vi "Parse NT String Array.vi"(11 "TCP Network Connection in":refnum<k5>) -> (1 "Size":i32=1, 2 "String Array":string[](array[string]), 3 "TCP Network Connection out":refnum<k5>)   [LabVIEW 2017]
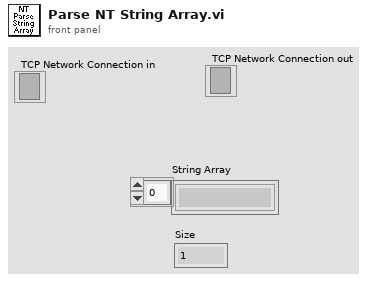
[diagram p1: front panel]
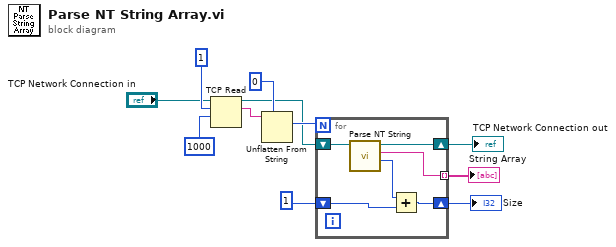
[diagram p0: block diagram]
diagram:
  n1 = TCP Read(connection ID="TCP Network Connection in", bytes to read=1 ("timeout ms (25000)"), 9:1000 ("timeout ms (25000)")) -> (connection ID out=w5:refnum<k5>, data out=w8:string)  [unwired: 2 in, 1 out]
  n2 = Unflatten From String(type=u8 0 ("Size"), binary string=w8) -> (value=w6:u8)  [unwired: 3 in, 2 out]
  n3 = for {
    N: w6 -> [_]
    shift-right: [w16] -> w4
    shift-left: w5 -> [w17]
    tunnel: [w15] -> w3 mode=indexing
    shift-right: [w13] -> w1
    shift-left: 1 ("timeout ms (25000)") -> [w14]
    n4 = call <vilib>:"Parse NT String.vi"("TCP Network Connection in"=w17) -> ("Size"=w12:i32, "String"=w15:string, "TCP Network Connection out"=w16:refnum<k5>)  [unwired: 8 in]
    n5 = Add(x=w12, y=w14) -> (x+y=w13:i32)
  }
  "TCP Network Connection out" <- w4
  "String Array" <- w3
  "Size" <- w1
